vi "Build Custom VI Documentation Report.vi"(8 "error in (no error)":errorcluster, 9 "custom contents options":T1 {"list of controls options"."list which controls?" items=["all controls", "connected controls"]}, 10 "VI reference":refnum<vi>, 11 "report in":refnum<class "NI_report.lvclass">) -> (0 "error out":errorcluster, 3 "report out":refnum<class "NI_report.lvclass">)   [LabVIEW 2020, in "NI_ReportGenerationCore.lvlib"]
uses:
  <vilib>/Utility/NIReport.llb/NI_ReportGenerationCore.lvlib
  <vilib>/Utility/NIReport.llb/NI_report.lvclass
  <vilib>/printing/EasyPrintingControls.llb/custom_contents_options.ctl
  <vilib>/printing/EasyPrintingControls.llb/list_which_controls.ctl
panel:
  in  "Hierarchy section title":string="Position in Hierarchy"
  in  "History section title":string="History"
  in  "List of SubVIs section title":string="List of SubVIs"
  in  "Block Diagram section title":string="Block Diagram"
  in  "Controls section title":string="Controls and Indicators"
  in  "Front Panel section title":string="Front Panel"
  in  "Connector Pane section title":string="Connector Pane"
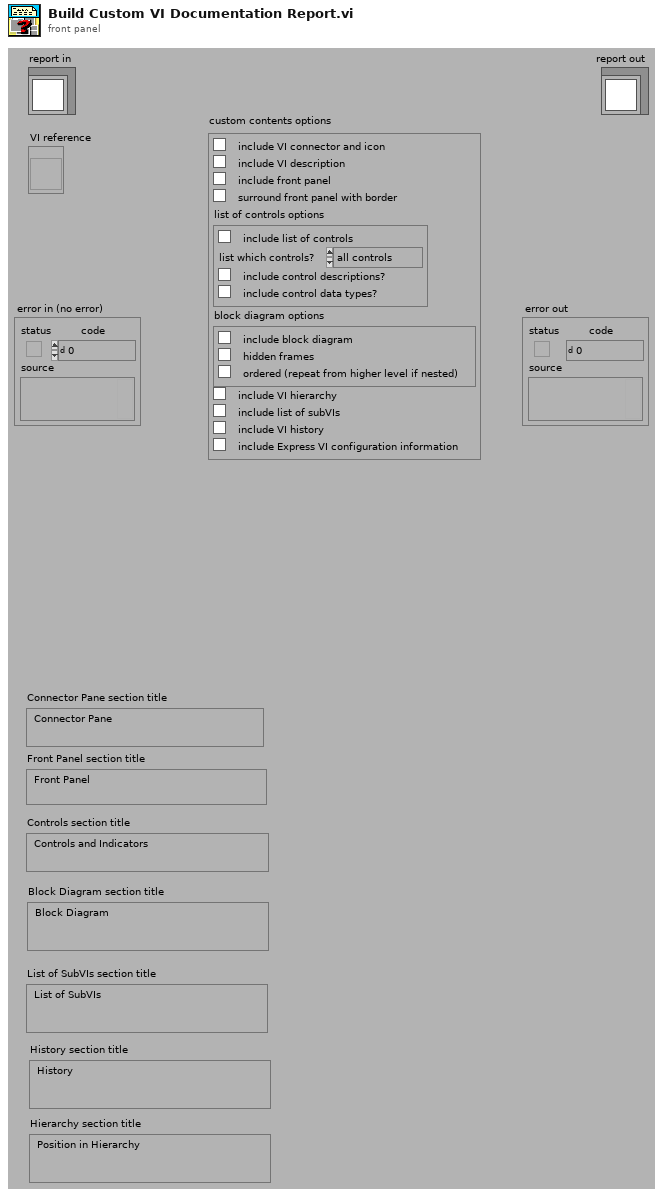
[diagram p1: front panel]
types:
  T1 = typedef "NI_ReportGenerationCore.lvlib/custom_contents_options.ctl" = cluster{"include VI connector and icon":bool, "include VI description":bool, "include front panel":bool, "surround front panel with border":bool, "list of controls options":cluster{"include list of controls":bool, "list which controls?":T2, "include control descriptions?":bool, "include control data types?":bool}, "block diagram options":cluster{"include block diagram":bool, "hidden frames":bool, "ordered (repeat from higher level if nested)":bool}, "include VI hierarchy":bool, "include list of subVIs":bool, "include VI history":bool, "include Express VI configuration information":bool}
  T2 = typedef "NI_ReportGenerationCore.lvlib/list_which_controls.ctl" = u16
  T3 = cluster{"position (excel)":cluster{"row":i32, "column":i32}, "name (excel)":string, "bookmark (word)":string}
  T4 = cluster{"position (Excel)":cluster{"row":i32, "column":i32}, "name (Excel)":string, "bookmark (Word)":string}
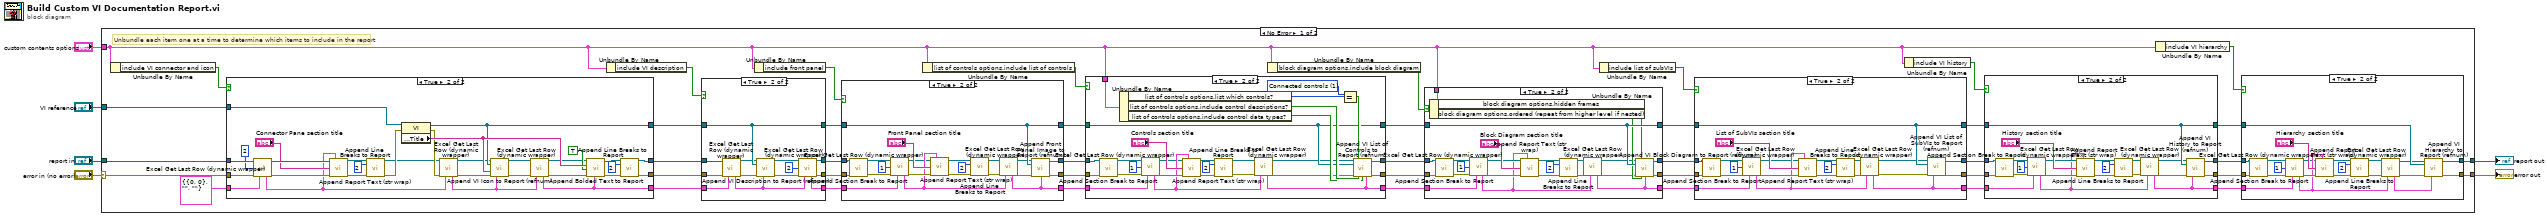
[diagram p0: block diagram]
diagram:
  n1 = case shown="No Error" "error in (no error)" {
    selector: "error in (no error)" -> [w7 w259]
    tunnel: "report in" -> [w49 w260]
    tunnel: "VI reference" -> [w48 _]
    tunnel: [w35 w260] -> w1
    tunnel: [w34 w259] -> w4
    tunnel: "custom contents options" -> [w8 _]
    frame No Error {
      # "Unbundle each item one at a time to determine which items to include in the report"
      n2 = Unbundle By Name(w8) -> ("include VI connector and icon"=w31:bool)
      n3 = case shown="True" w31 {
        tunnel: w7 -> [w200 w223]
        tunnel: w49 -> [w201 w222]
        tunnel: w48 -> [w202 w233]
        tunnel: [w202 w204] -> w29
        tunnel: [w200 w225] -> w33
        tunnel: [w201 w224] -> w32
        tunnel: T3 {"position (excel)"={"row"=0, "column"=0}, "name (excel)"="", "bookmark (word)"=""} ("MS Office parameters") -> [w199 w213]
        tunnel: [w199 w211] -> w15
        frame False {
        }
        frame True {
          n4 = call <vilib>:"Excel Get Last Row (dynamic wrapper).vi"("report in"=w222, "offset"=2, "error in (no error)"=w223, "MS Office parameters"=w213) -> ("report out"=w210:refnum<class "NI_report.lvclass">, "MS Office parameters out"=w205:T4, "error out"=w209:errorcluster)  [unwired: 9 in]
          n5 = call <vilib>:"Append Report Text (str wrap).vi"("report in"=w210, "MS Office parameters"=w205, "text"="Connector Pane section title", "error in (no error)"=w209) -> ("report out"=w207:refnum<class "NI_report.lvclass">, "error out"=w206:errorcluster)  [unwired: 8 in, 2 out]
          n6 = call <vilib>:"Append Line Breaks to Report.vi"("report in"=w207, "number of line breaks"=u32 2 ("Number of line breaks"), "error in (no error)"=w206) -> ("report out"=w219:refnum<class "NI_report.lvclass">, "error out"=w232:errorcluster)  [unwired: 11 in]
          n7 = property class="VI"(reference=w233, error in=w232) -> (reference out=w204:refnum<vi>, error out=w221:errorcluster, "Front Panel Window:Title"=w230:string)
          n8 = call <vilib>:"Excel Get Last Row (dynamic wrapper).vi"("report in"=w219, "error in (no error)"=w221, "MS Office parameters"=w205) -> ("report out"=w203:refnum<class "NI_report.lvclass">, "MS Office parameters out"=w212:T4, "error out"=w220:errorcluster)  [unwired: 10 in]
          n9 = call <vilib>:"Append VI Icon to Report (refnum).vi"("report in"=w203, "VI"=w204, "caption or alternative string"=w230, "error in (no error)"=w220, "MS Office parameters"=w212) -> ("report out"=w218:refnum<class "NI_report.lvclass">, "error out"=w215:errorcluster)  [unwired: 6 in, 3 out]
          n10 = call <vilib>:"Excel Get Last Row (dynamic wrapper).vi"("report in"=w218, "error in (no error)"=w215, "MS Office parameters"=w212) -> ("report out"=w217:refnum<class "NI_report.lvclass">, "MS Office parameters out"=w211:T4, "error out"=w216:errorcluster)  [unwired: 10 in]
          n11 = call <vilib>:"Append Bolded Text to Report.vi"("MS Office parameters"=w211, "error in"=w216, "On new line?"=TRUE, "Text"=w230, "report in"=w217) -> ("error out"=w228:errorcluster, "report out"=w227:refnum<class "NI_report.lvclass">)  [unwired: 2 out]
          n12 = call <vilib>:"Append Line Breaks to Report.vi"("report in"=w227, "number of line breaks"=u32 2 ("Number of line breaks"), "error in (no error)"=w228) -> ("report out"=w224:refnum<class "NI_report.lvclass">, "error out"=w225:errorcluster)  [unwired: 11 in]
        }
      }
      n13 = Unbundle By Name(w8) -> ("include VI description"=w30:bool)
      n14 = case shown="True" w30 {
        tunnel: [w183 w191] -> w47
        tunnel: [w184 w192] -> w46
        tunnel: w29 -> [w185 w198]
        tunnel: w33 -> [w183 w197]
        tunnel: w32 -> [w184 w196]
        tunnel: [w185 w198] -> w28
        tunnel: w15 -> [w182 w194]
        tunnel: [w182 w188] -> w14
        frame False {
        }
        frame True {
          n15 = call <vilib>:"Excel Get Last Row (dynamic wrapper).vi"("report in"=w196, "error in (no error)"=w197, "MS Office parameters"=w194) -> ("report out"=w186:refnum<class "NI_report.lvclass">, "MS Office parameters out"=w189:T4, "error out"=w195:errorcluster)  [unwired: 10 in]
          n16 = call <vilib>:"Append VI Description to Report (refnum).vi"("report in"=w186, "VI"=w198, "error in (no error)"=w195, "MS Office parameters"=w189) -> ("report out"=w193:refnum<class "NI_report.lvclass">, "error out"=w190:errorcluster)  [unwired: 7 in, 3 out]
          n17 = call <vilib>:"Excel Get Last Row (dynamic wrapper).vi"("report in"=w193, "offset"=2, "error in (no error)"=w190, "MS Office parameters"=w189) -> ("report out"=w192:refnum<class "NI_report.lvclass">, "MS Office parameters out"=w188:T4, "error out"=w191:errorcluster)  [unwired: 9 in]
        }
      }
      n18 = Unbundle By Name(w8) -> ("include front panel"=w27:bool)
      n19 = case shown="True" w27 {
        tunnel: w47 -> [w235 w258]
        tunnel: w46 -> [w236 w257]
        tunnel: [w235 w256] -> w45
        tunnel: [w236 w255] -> w44
        tunnel: w28 -> [w237 w253]
        tunnel: [w237 w253] -> w26
        tunnel: w14 -> [w234 w246]
        tunnel: [w234 w245] -> w13
        frame False {
        }
        frame True {
          n20 = call-dynamic "Append Section Break to Report.vi"("report in"=w257, "error in (no error)"=w258) -> ("report out"=w252:refnum<class "NI_report.lvclass">, "error out"=w251:errorcluster)  [unwired: 12 in]
          n21 = call <vilib>:"Excel Get Last Row (dynamic wrapper).vi"("report in"=w252, "offset"=1, "error in (no error)"=w251, "MS Office parameters"=w246) -> ("report out"=w241:refnum<class "NI_report.lvclass">, "MS Office parameters out"=w242:T4, "error out"=w244:errorcluster)  [unwired: 9 in]
          n22 = call <vilib>:"Append Report Text (str wrap).vi"("report in"=w241, "MS Office parameters"=w242, "text"="Front Panel section title", "error in (no error)"=w244) -> ("report out"=w239:refnum<class "NI_report.lvclass">, "error out"=w240:errorcluster)  [unwired: 8 in, 2 out]
          n23 = call <vilib>:"Append Line Breaks to Report.vi"("report in"=w239, "number of line breaks"=u32 2 ("Number of line breaks"), "error in (no error)"=w240) -> ("report out"=w248:refnum<class "NI_report.lvclass">, "error out"=w250:errorcluster)  [unwired: 11 in]
          n24 = call <vilib>:"Excel Get Last Row (dynamic wrapper).vi"("report in"=w248, "error in (no error)"=w250, "MS Office parameters"=w242) -> ("report out"=w238:refnum<class "NI_report.lvclass">, "MS Office parameters out"=w245:T4, "error out"=w249:errorcluster)  [unwired: 10 in]
          n25 = call <vilib>:"Append Front Panel Image to Report (refnum).vi"("report in"=w238, "VI"=w253, "error in (no error)"=w249, "MS Office parameters"=w245) -> ("report out"=w255:refnum<class "NI_report.lvclass">, "error out"=w256:errorcluster)  [unwired: 7 in, 3 out]
        }
      }
      n26 = Unbundle By Name(w8) -> ("list of controls options.include list of controls"=w25:bool)
      n27 = case shown="True" w25 {
        tunnel: w45 -> [w152 w181]
        tunnel: w44 -> [w153 w180]
        tunnel: [w153 w178] -> w43
        tunnel: [w152 w177] -> w42
        tunnel: w26 -> [w154 w170]
        tunnel: w8 -> [_ w176]
        tunnel: [w154 w170] -> w24
        tunnel: w13 -> [w151 w164]
        tunnel: [w151 w162] -> w12
        frame False {
        }
        frame True {
          w175 = T2 1 items=["All controls", "Connected controls"] ("list of controls options.List which controls?")
          n28 = call-dynamic "Append Section Break to Report.vi"("report in"=w180, "error in (no error)"=w181) -> ("report out"=w169:refnum<class "NI_report.lvclass">, "error out"=w168:errorcluster)  [unwired: 12 in]
          n29 = Unbundle By Name(w176) -> ("list of controls options.list which controls?"=w174:T2, "list of controls options.include control descriptions?"=w172:bool, "list of controls options.include control data types?"=w171:bool)
          n30 = call <vilib>:"Excel Get Last Row (dynamic wrapper).vi"("report in"=w169, "offset"=1, "error in (no error)"=w168, "MS Office parameters"=w164) -> ("report out"=w156:refnum<class "NI_report.lvclass">, "MS Office parameters out"=w157:T4, "error out"=w158:errorcluster)  [unwired: 9 in]
          n31 = call <vilib>:"Append Report Text (str wrap).vi"("report in"=w156, "MS Office parameters"=w157, "text"="Controls section title", "error in (no error)"=w158) -> ("report out"=w161:refnum<class "NI_report.lvclass">, "error out"=w160:errorcluster)  [unwired: 8 in, 2 out]
          n32 = call <vilib>:"Append Line Breaks to Report.vi"("report in"=w161, "number of line breaks"=u32 2 ("Number of line breaks"), "error in (no error)"=w160) -> ("report out"=w167:refnum<class "NI_report.lvclass">, "error out"=w166:errorcluster)  [unwired: 11 in]
          n33 = call <vilib>:"Excel Get Last Row (dynamic wrapper).vi"("report in"=w167, "error in (no error)"=w166, "MS Office parameters"=w157) -> ("report out"=w155:refnum<class "NI_report.lvclass">, "MS Office parameters out"=w162:T4, "error out"=w165:errorcluster)  [unwired: 10 in]
          n34 = Equal?(x=w175, y=w174) -> (x = y?=w173:bool)
          n35 = call <vilib>:"Append VI List of Controls to Report (refnum).vi"("report in"=w155, "include only controls in con pane?"=w173, "VI"=w170, "error in (no error)"=w165, "include control descriptions?"=w172, "include control data types?"=w171, "MS Office parameters"=w162) -> ("report out"=w178:refnum<class "NI_report.lvclass">, "error out"=w177:errorcluster)  [unwired: 4 in, 3 out]
        }
      }
      n36 = Unbundle By Name(w8) -> ("block diagram options.include block diagram"=w22:bool)
      n37 = case shown="True" w22 {
        tunnel: w43 -> [w125 w150]
        tunnel: w42 -> [w124 w149]
        tunnel: [w125 w147] -> w41
        tunnel: [w124 w146] -> w40
        tunnel: w24 -> [w126 w145]
        tunnel: [w126 w145] -> w23
        tunnel: w12 -> [w123 w137]
        tunnel: [w123 w135] -> w11
        tunnel: w8 -> [_ w134]
        frame False {
        }
        frame True {
          n38 = Unbundle By Name(w134) -> ("block diagram options.hidden frames"=w144:bool, "block diagram options.ordered (repeat from higher level if nested)"=w143:bool)
          n39 = call-dynamic "Append Section Break to Report.vi"("report in"=w150, "error in (no error)"=w149) -> ("report out"=w142:refnum<class "NI_report.lvclass">, "error out"=w141:errorcluster)  [unwired: 12 in]
          n40 = call <vilib>:"Excel Get Last Row (dynamic wrapper).vi"("report in"=w142, "offset"=1, "error in (no error)"=w141, "MS Office parameters"=w137) -> ("report out"=w129:refnum<class "NI_report.lvclass">, "MS Office parameters out"=w128:T4, "error out"=w130:errorcluster)  [unwired: 9 in]
          n41 = call <vilib>:"Append Report Text (str wrap).vi"("report in"=w129, "MS Office parameters"=w128, "text"="Block Diagram section title", "error in (no error)"=w130) -> ("report out"=w132:refnum<class "NI_report.lvclass">, "error out"=w133:errorcluster)  [unwired: 8 in, 2 out]
          n42 = call <vilib>:"Append Line Breaks to Report.vi"("report in"=w132, "number of line breaks"=u32 2 ("Number of line breaks"), "error in (no error)"=w133) -> ("report out"=w140:refnum<class "NI_report.lvclass">, "error out"=w139:errorcluster)  [unwired: 11 in]
          n43 = call <vilib>:"Excel Get Last Row (dynamic wrapper).vi"("report in"=w140, "error in (no error)"=w139, "MS Office parameters"=w128) -> ("report out"=w127:refnum<class "NI_report.lvclass">, "MS Office parameters out"=w135:T4, "error out"=w138:errorcluster)  [unwired: 10 in]
          n44 = call <vilib>:"Append VI Block Diagram to Report (refnum).vi"("report in"=w127, "hidden frames"=w144, "VI"=w145, "error in (no error)"=w138, "ordered (repeat from higher level if nested)"=w143, "MS Office parameters"=w135) -> ("report out"=w147:refnum<class "NI_report.lvclass">, "error out"=w146:errorcluster)  [unwired: 5 in, 3 out]
        }
      }
      n45 = Unbundle By Name(w8) -> ("include list of subVIs"=w21:bool)
      n46 = case shown="True" w21 {
        tunnel: w41 -> [w100 w122]
        tunnel: w40 -> [w99 w121]
        tunnel: [w99 w119] -> w39
        tunnel: [w100 w118] -> w38
        tunnel: w23 -> [w101 w117]
        tunnel: [w101 w117] -> w20
        tunnel: w11 -> [w98 w110]
        tunnel: [w98 w109] -> w10
        frame False {
        }
        frame True {
          n47 = call-dynamic "Append Section Break to Report.vi"("report in"=w122, "error in (no error)"=w121) -> ("report out"=w115:refnum<class "NI_report.lvclass">, "error out"=w116:errorcluster)  [unwired: 12 in]
          n48 = call <vilib>:"Excel Get Last Row (dynamic wrapper).vi"("report in"=w115, "offset"=1, "error in (no error)"=w116, "MS Office parameters"=w110) -> ("report out"=w103:refnum<class "NI_report.lvclass">, "MS Office parameters out"=w104:T4, "error out"=w106:errorcluster)  [unwired: 9 in]
          n49 = call <vilib>:"Append Report Text (str wrap).vi"("report in"=w103, "MS Office parameters"=w104, "text"="List of SubVIs section title", "error in (no error)"=w106) -> ("report out"=w107:refnum<class "NI_report.lvclass">, "error out"=w108:errorcluster)  [unwired: 8 in, 2 out]
          n50 = call <vilib>:"Append Line Breaks to Report.vi"("report in"=w107, "number of line breaks"=u32 2 ("Number of line breaks"), "error in (no error)"=w108) -> ("report out"=w112:refnum<class "NI_report.lvclass">, "error out"=w114:errorcluster)  [unwired: 11 in]
          n51 = call <vilib>:"Excel Get Last Row (dynamic wrapper).vi"("report in"=w112, "error in (no error)"=w114, "MS Office parameters"=w104) -> ("report out"=w102:refnum<class "NI_report.lvclass">, "MS Office parameters out"=w109:T4, "error out"=w113:errorcluster)  [unwired: 10 in]
          n52 = call <vilib>:"Append VI List of SubVIs to Report (refnum).vi"("report in"=w102, "VI"=w117, "error in (no error)"=w113, "MS Office parameters"=w109) -> ("report out"=w118:refnum<class "NI_report.lvclass">, "error out"=w119:errorcluster)  [unwired: 7 in, 3 out]
        }
      }
      n53 = Unbundle By Name(w8) -> ("include VI history"=w19:bool)
      n54 = case shown="True" w19 {
        tunnel: w39 -> [w74 w97]
        tunnel: w38 -> [w75 w96]
        tunnel: [w74 w94] -> w37
        tunnel: [w75 w93] -> w36
        tunnel: w20 -> [w76 w92]
        tunnel: [w76 w92] -> w18
        tunnel: w10 -> [w73 w85]
        tunnel: [w73 w84] -> w9
        frame False {
        }
        frame True {
          n55 = call-dynamic "Append Section Break to Report.vi"("report in"=w96, "error in (no error)"=w97) -> ("report out"=w87:refnum<class "NI_report.lvclass">, "error out"=w88:errorcluster)  [unwired: 12 in]
          n56 = call <vilib>:"Excel Get Last Row (dynamic wrapper).vi"("report in"=w87, "offset"=1, "error in (no error)"=w88, "MS Office parameters"=w85) -> ("report out"=w79:refnum<class "NI_report.lvclass">, "MS Office parameters out"=w77:T4, "error out"=w81:errorcluster)  [unwired: 9 in]
          n57 = call <vilib>:"Append Report Text (str wrap).vi"("report in"=w79, "MS Office parameters"=w77, "text"="History section title", "error in (no error)"=w81) -> ("report out"=w83:refnum<class "NI_report.lvclass">, "error out"=w82:errorcluster)  [unwired: 8 in, 2 out]
          n58 = call <vilib>:"Append Line Breaks to Report.vi"("report in"=w83, "number of line breaks"=u32 2 ("Number of line breaks"), "error in (no error)"=w82) -> ("report out"=w91:refnum<class "NI_report.lvclass">, "error out"=w90:errorcluster)  [unwired: 11 in]
          n59 = call <vilib>:"Excel Get Last Row (dynamic wrapper).vi"("report in"=w91, "error in (no error)"=w90, "MS Office parameters"=w77) -> ("report out"=w78:refnum<class "NI_report.lvclass">, "MS Office parameters out"=w84:T4, "error out"=w89:errorcluster)  [unwired: 10 in]
          n60 = call <vilib>:"Append VI History to Report (refnum).vi"("report in"=w78, "VI"=w92, "error in (no error)"=w89, "MS Office parameters"=w84) -> ("report out"=w93:refnum<class "NI_report.lvclass">, "error out"=w94:errorcluster)  [unwired: 7 in, 3 out]
        }
      }
      n61 = Unbundle By Name(w8) -> ("include VI hierarchy"=w17:bool)
      n62 = case shown="True" w17 {
        tunnel: w37 -> [w50 w72]
        tunnel: w36 -> [w51 w71]
        tunnel: [w51 w69] -> w35
        tunnel: [w50 w68] -> w34
        tunnel: w18 -> [_ w67]
        tunnel: w9 -> [_ w59]
        frame False {
        }
        frame True {
          n63 = call-dynamic "Append Section Break to Report.vi"("report in"=w71, "error in (no error)"=w72) -> ("report out"=w66:refnum<class "NI_report.lvclass">, "error out"=w65:errorcluster)  [unwired: 12 in]
          n64 = call <vilib>:"Excel Get Last Row (dynamic wrapper).vi"("report in"=w66, "offset"=1, "error in (no error)"=w65, "MS Office parameters"=w59) -> ("report out"=w52:refnum<class "NI_report.lvclass">, "MS Office parameters out"=w53:T4, "error out"=w57:errorcluster)  [unwired: 9 in]
          n65 = call <vilib>:"Append Report Text (str wrap).vi"("report in"=w52, "MS Office parameters"=w53, "text"="Hierarchy section title", "error in (no error)"=w57) -> ("report out"=w55:refnum<class "NI_report.lvclass">, "error out"=w56:errorcluster)  [unwired: 8 in, 2 out]
          n66 = call <vilib>:"Append Line Breaks to Report.vi"("report in"=w55, "number of line breaks"=u32 2 ("Number of line breaks"), "error in (no error)"=w56) -> ("report out"=w64:refnum<class "NI_report.lvclass">, "error out"=w63:errorcluster)  [unwired: 11 in]
          n67 = call <vilib>:"Excel Get Last Row (dynamic wrapper).vi"("report in"=w64, "error in (no error)"=w63, "MS Office parameters"=w53) -> ("report out"=w61:refnum<class "NI_report.lvclass">, "MS Office parameters out"=w58:T4, "error out"=w62:errorcluster)  [unwired: 10 in]
          n68 = call <vilib>:"Append VI Hierarchy to Report (refnum).vi"("report in"=w61, "VI"=w67, "error in (no error)"=w62, "MS Office parameters"=w58) -> ("report out"=w69:refnum<class "NI_report.lvclass">, "error out"=w68:errorcluster)  [unwired: 7 in, 3 out]
        }
      }
    }
    frame Error {
    }
  }
  "report out" <- w1
  "error out" <- w4
